vi "LlenarVoltajeTabla.vi"(7 "Frecuencia":string, 10 "Dato":string, 11 "Tabla in":string[][](array[string])) -> (3 "Tabla out":string[][](array[string]))   [LabVIEW 2019, in "Prueba33.lvclass"]
uses:
  Prueba33.lvclass
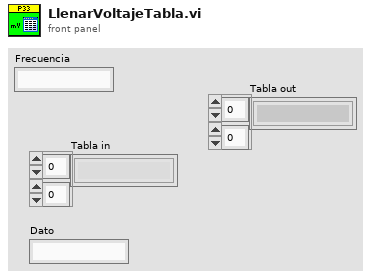
[diagram p1: front panel]
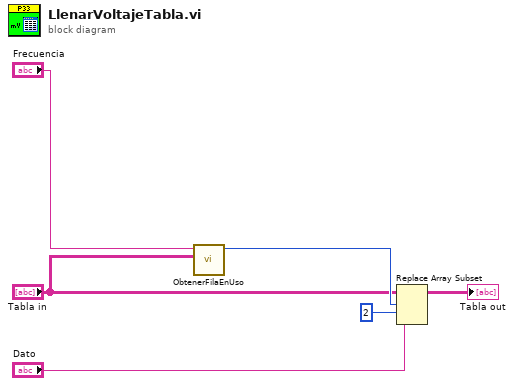
[diagram p0: block diagram]
diagram:
  n1 = call "ObtenerFilaEnUso.vi"("Tabla in"="Tabla in", "Frecuencia"="Frecuencia") -> ("index of element"=w3:i32)  [unwired: 9 in]
  n2 = Replace Array Subset(array="Tabla in", new element="Dato", index (row)=w3, index (col)=2 ("disabled index (col)")) -> (→"Tabla out":string[][])
